vi "SalcompMESSaveResultXML).vi"(10 "XmlFileContent":string) -> (2 "SaveResult":bool)   [LabVIEW 2018]
uses:
  CMESAPI.dll
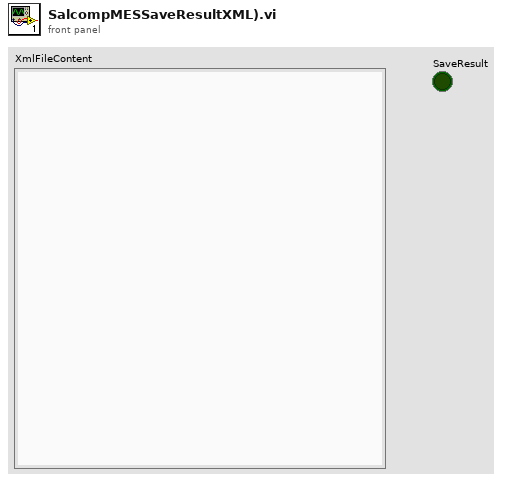
[diagram p1: front panel]
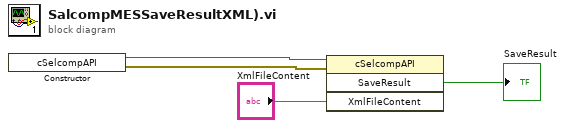
[diagram p0: block diagram]
diagram:
  n1 = constructor class="cSelcompAPI"() -> (reference out=w4:refnum<k24>, error out=w3:errorcluster)  [unwired: 3 in, 1 out]
  n2 = invoke class="cSelcompAPI" method="SaveResult"(reference=w4, error in=w3, "XmlFileContent"="XmlFileContent") -> ("SaveResult"=→"SaveResult":bool)  [unwired: 1 in, 3 out]
